vi "Cleanup Channels.vi"(8 "error in (no error)":errorcluster, 11 "Plugin In":refnum<class "Sequencer with Output Values.lvclass">) -> (0 "error out":errorcluster, 1 "Num of Digital Channels":i32, 2 "Num of Analog Channels":i32, 3 "Plugin out":refnum<class "Sequencer with Output Values.lvclass">)   [LabVIEW 2024, in "Sequencer with Output Values.lvlib" / "Sequencer with Output Values.lvclass"]
uses:
  Sequencer with Output Values.lvclass
  C:/Program Files/National Instruments/LabVIEW 2024/vi.lib/FlexLogger/SDK/PluginSDK.lvlibp/PEFClasses/SDK/Plugin/Plugin.lvclass
  <vilib>/FlexLogger/SDK/PluginSDK.lvlibp/PEFClasses/SDK/Channel/Data Type_v2.ctl
  Sequencer with Output Values.lvclass/Sequencer with Output Values.ctl
  Global Strings.vi
  <vilib>/FlexLogger/SDK/PluginSDK.lvlibp/PEFClasses/SDK/Plugin/Read Channels.vi
  <vilib>/FlexLogger/SDK/PluginSDK.lvlibp/PEFClasses/SDK/Channel/Channel.lvclass
  <vilib>/FlexLogger/SDK/PluginSDK.lvlibp
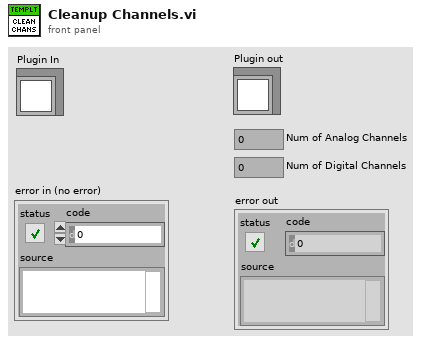
[diagram p1: front panel]
types:
  T1 = typedef "PluginSDK.lvlibp/Channel.lvclass/Data Type_v2.ctl" = u16
  T2 = typedef "Sequencer with Output Values.lvlib/Sequencer with Output Values.lvclass/Params.ctl" = cluster{"Step Values":T3[], "Only Execute When Test Running":bool, "Reset Sequence When Test Starts":bool, "Current Sequence ID":u32, "Total Iterations":u32, "Current Step Start Timestamp":dbl, "Number of Sequence Steps":i32, "Num of Analog Channels":i32, "Num of Digital Channels":i32, "Delay Before Starting Sequence":dbl, "Show UI":bool, "Time Remaining":dbl, "Test Running":bool, "Pause Timestamp":dbl}
  T3 = typedef "Sequencer with Output Values.lvlib/Sequencer with Output Values.lvclass/Step Settings.ctl" = cluster{"Duration":dbl, "Mode":string, "Delay Between Values":dbl, "Analog Values":string[], "Digital Values":string[]}
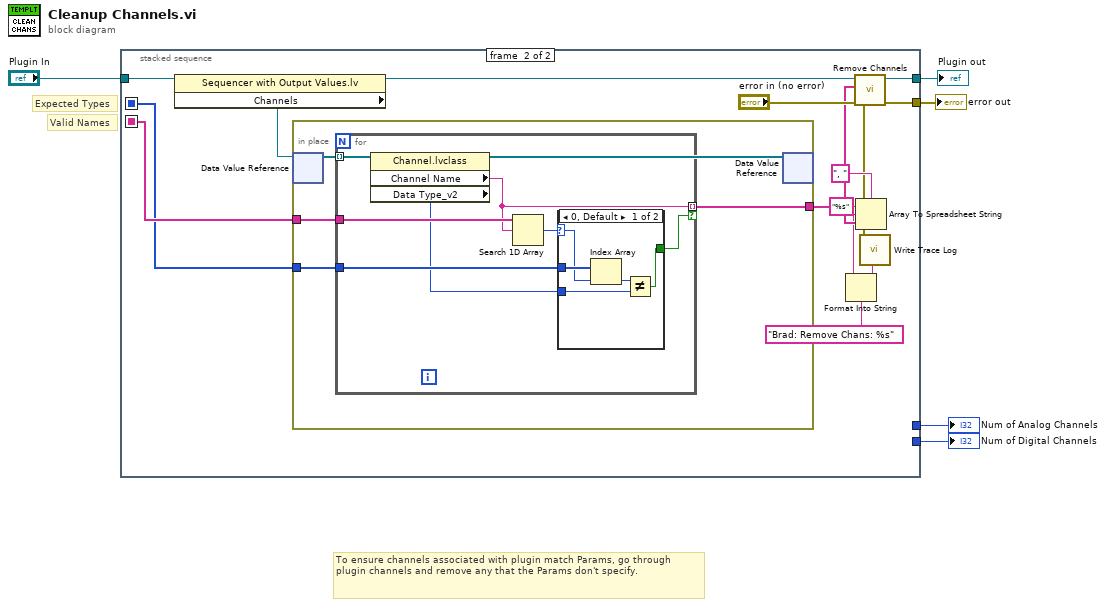
[diagram p0: block diagram]
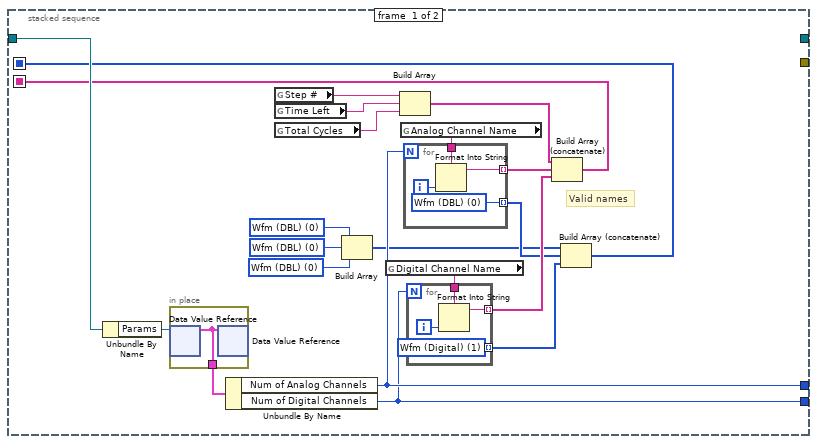
[diagram p2: hidden frame]
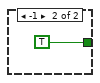
[diagram p3: hidden frame]
diagram:
  # "Expected Types"
  # "Valid Names"
  # "To ensure channels associated with plugin match Params, go through plugin channels and remove any that the Params don't specify."
  n1 = stacked-sequence {
    seq-local: [w19 _] -> [_ w46]
    seq-local: [w6 _] -> [_ w36]
    tunnel: [w18 _] -> w5
    tunnel: "Plugin In" -> [w26 w47]
    tunnel: [w23 _] -> w3
    tunnel: [_ w37] -> w2
    tunnel: [_ w44] -> w1
    frame #0 {
      w9 = T1 0 items=["Wfm (DBL)", "Wfm (Digital)", "String"] ("Data Type_v2")
      w10 = T1 0 items=["Wfm (DBL)", "Wfm (Digital)", "String"] ("Data Type_v2")
      w11 = T1 0 items=["Wfm (DBL)", "Wfm (Digital)", "String"] ("Data Type_v2")
      # "Valid names"
      n2 = Unbundle By Name(w26) -> ("Params"=w24:refnum<data-value>)
      n3 = in-place {
        in-place-border: [w35] -> w25
        n4 = in-place-dvr #1(w24) -> (w35:T2)  [unwired: 1 out]
        n5 = in-place-dvr #1(w35) -> ()  [unwired: 2 out]
      }
      n6 = Unbundle By Name(w25) -> ("Num of Analog Channels"=w23:i32, "Num of Digital Channels"=w18:i32)
      n7 = global read "Global Strings.vi" "Step #"() -> (w17:string)
      n8 = global read "Global Strings.vi" "Time Left"() -> (w16:string)
      n9 = global read "Global Strings.vi" "Total Cycles"() -> (w15:string)
      n10 = Build Array(w11, w10, w9) -> (w8:T1[])
      n11 = global read "Global Strings.vi" "Digital Channel Name"() -> (w21:string)
      n12 = Build Array(w17, w16, w15) -> (w14:string[])
      n13 = global read "Global Strings.vi" "Analog Channel Name"() -> (w22:string)
      n14 = for {
        N: w23 -> [_]
        tunnel: w22 -> [w33]
        tunnel: [w32] -> w20 mode=indexing
        tunnel: [w31] -> w12 mode=indexing
        i -> [w34]
        w31 = T1 0 items=["Wfm (DBL)", "Wfm (Digital)", "String"] ("Data Type_v2")
        n15 = Format Into String(format string=w33, w34) -> (resulting string=w32:string)  [unwired: 2 in, 1 out]
      }
      n16 = for {
        N: w18 -> [_]
        tunnel: w21 -> [w29]
        tunnel: [w28] -> w13 mode=indexing
        tunnel: [w27] -> w7 mode=indexing
        i -> [w30]
        w27 = T1 1 items=["Wfm (DBL)", "Wfm (Digital)", "String"] ("Data Type_v2")
        n17 = Format Into String(format string=w29, w30) -> (resulting string=w28:string)  [unwired: 2 in, 1 out]
      }
      n18 = Build Array (concatenate)(w14, w20, w13) -> (w19:string[])
      n19 = Build Array (concatenate)(w8, w12, w7) -> (w6:T1[])
    }
    frame #1 {
      n20 = property class="Sequencer with Output Values.lv"(reference=w47) -> (reference out=w49:refnum<class "Sequencer with Output Values.lvclass">, "Channels"=w48:refnum<data-value>)  [unwired: 1 in, 1 out]
      n21 = in-place {
        in-place-border: [w52] -> w42
        in-place-border: w46 -> [w51]
        in-place-border: w36 -> [w50]
        n22 = in-place-dvr #2(w48) -> (w53:refnum<class "Channel.lvclass">[])  [unwired: 1 out]
        n23 = for {
          tunnel: w53 -> [w60] mode=indexing
          tunnel: [w58] -> w52 mode=indexing if=w56
          tunnel: w51 -> [w59]
          tunnel: w50 -> [w55]
          n24 = property class="Channel.lvclass"(reference=w60) -> ("Channel Name"=w58:string, "Data Type_v2"=w54:T1)  [unwired: 1 in, 2 out]
          n25 = Search 1D Array(1D array=w59, element=w58) -> (index of element=w57:i32)  [unwired: 1 in]
          n26 = case shown="0, Default" w57 {
            selector: w57 -> [w64 _]
            tunnel: [w61 TRUE] -> w56
            tunnel: w55 -> [w65 _]
            tunnel: w54 -> [w62 _]
            frame 0, Default {
              n27 = Index Array(array=w65, index=w64) -> (element=w63:T1)
              n28 = Not Equal?(x=w63, y=w62) -> (x != y?=w61:bool)
            }
            frame -1 {
            }
          }
        }
        n29 = in-place-dvr #2(w53) -> ()  [unwired: 2 out]
      }
      n30 = call-dynamic "Remove Channels.vi"("error in (no error)"="error in (no error)", "Unique Channel Identifiers to Delete"=w42, "Plugin in"=w49) -> ("error out"=w37:errorcluster, "Plugin out"=w44:refnum<class "Sequencer with Output Values.lvclass">)  [unwired: 7 in]
      n31 = Array To Spreadsheet String(delimiter (Tab)=", ", array=w42, 3:"%s" ("format string")) -> (spreadsheet string=w39:string)
      n32 = Format Into String(format string="Brad: Remove Chans: %s", w39) -> (resulting string=w38:string)  [unwired: 2 in, 1 out]
      n33 = call <vilib>:"Write Trace Log.vi"("error in (no error)"=w37, "Message"=w38) -> ()  [unwired: 9 in, 1 out]
    }
  }
  "Num of Analog Channels" <- w3
  "Num of Digital Channels" <- w5
  "error out" <- w2
  "Plugin out" <- w1
